vi "read command.vi"(9 "timeout ms (25000)":i32=25000) -> (0 "error out":errorcluster, 1 "command received":bool, 2 "command interface":T1={"command"=enum."Idle", "start time (ms)"=0, "Channel Indices"=[], "Scans per Sample"=1} {"Scans per Sample" min=1})   [LabVIEW 2012]
uses:
  DataServer/command cluster.ctl
  DataServer/command.ctl
panel:
  out "bytes read":dbl format="%.2f"
  out "byte received":bool
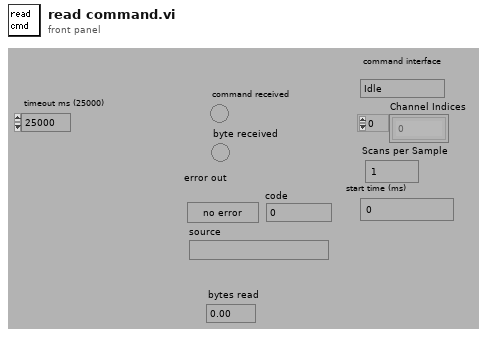
[diagram p1: front panel]
types:
  T1 = typedef "command cluster.ctl" = cluster{"command":T2, "start time (ms)":u32, "Channel Indices":i32[], "Scans per Sample":i32}
  T2 = typedef "command.ctl" = enum16{"Idle", "Send Data", "Send 1 Scan", "Logoff"}
  T3 = enum16{"clear", "add connection", "change command", "write state", "delete connection", "read"}
  T4 = enum16{"Standard", "Buffered", "CRLF", "Immediate"}
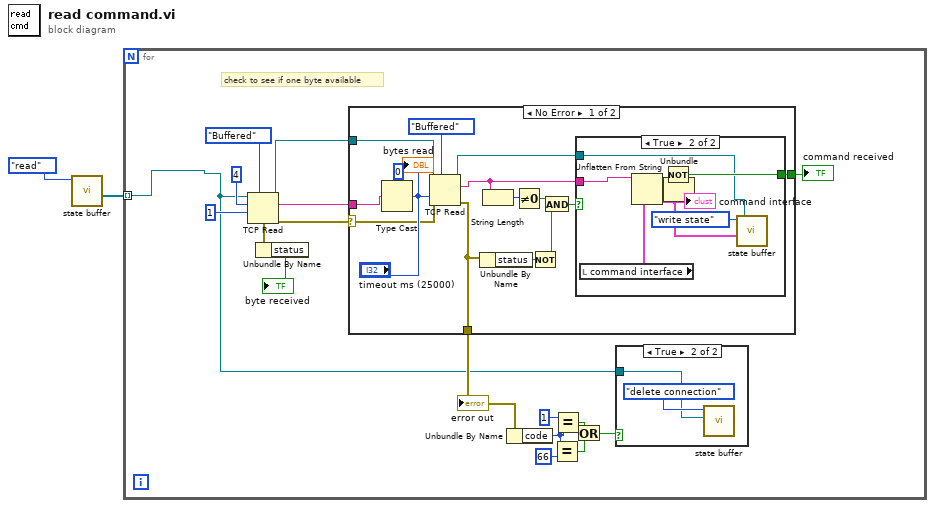
[diagram p0: block diagram]
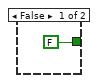
[diagram p3: hidden frame]
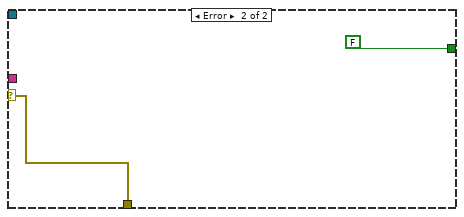
[diagram p4: hidden frame]
diagram:
  n1 = call "state buffer.vi"("command"=T3."read") -> ("connections"=w1:refnum<k5>[])  [unwired: 8 in, 2 out]
  n2 = for {
    tunnel: w1 -> [w4] mode=indexing
    # "check to see if one byte available"
    n3 = TCP Read(connection ID=w4, bytes to read=4, 7:T4."Buffered" ("mode (standard)"), 9:1) -> (connection ID out=w15:refnum<k5>, data out=w17:string, error out=w5:errorcluster)  [unwired: 1 in]
    n4 = Unbundle By Name(w5) -> ("status"=→"byte received":bool)
    n5 = case shown="No Error" w5 {
      selector: w5 -> [w22 w46]
      tunnel: w15 -> [w36 _]
      tunnel: w17 -> [w25 _]
      tunnel: [w23 w46] -> w12
      tunnel: [w27 FALSE] -> w14
      frame No Error {
        n6 = Type Cast(type=0, x=w25) -> (*(type *) &x=w26:i32)
        "bytes read" <- w26
        n7 = TCP Read(connection ID=w36, bytes to read=w26, error in (no error)=w22, 7:T4."Buffered" ("mode (standard)"), 9:"timeout ms (25000)") -> (connection ID out=w24:refnum<k5>, data out=w29:string, error out=w23:errorcluster)
        n8 = Unbundle By Name(w23) -> ("status"=w31:bool)
        n9 = String Length(string=w29) -> (length=w30:i32)
        n10 = Not Equal To 0?(x=w30) -> (x != 0?=w32:bool)
        n11 = Not(x=w31) -> (.not. x?=w33:bool)
        n12 = And(x=w32, y=w33) -> (x .and. y?=w28:bool)
        n13 = case shown="True" w28 {
          tunnel: w29 -> [_ w44]
          tunnel: [FALSE w42] -> w27
          tunnel: w24 -> [_ w40]
          frame False {
          }
          frame True {
            n14 = local read "command interface"() -> (w45:T1)
            n15 = Unflatten From String(type=w45, binary string=w44) -> (value=w39:T1, error out=w38:errorcluster)  [unwired: 3 in, 1 out]
            "command interface" <- w39
            n16 = Unbundle(w38) -> ("status"=w43:bool)  [unwired: 2 out]
            n17 = Not(x=w43) -> (.not. x?=w42:bool)
            n18 = call "state buffer.vi"("write state"=w39, "connection"=w40, "command"=T3."write state") -> ()  [unwired: 6 in, 3 out]
          }
        }
      }
      frame Error {
      }
    }
    "error out" <- w12
    "command received" <- w14
    n19 = Unbundle By Name(w12) -> ("code"=w11:i32)
    n20 = Equal?(x=w11, y=66) -> (x = y?=w8:bool)
    n21 = Equal?(x=1, y=w11) -> (x = y?=w9:bool)
    n22 = Or(x=w9, y=w8) -> (x .or. y?=w7:bool)
    n23 = case shown="True" w7 {
      tunnel: w4 -> [_ w19]
      frame False {
      }
      frame True {
        n24 = call "state buffer.vi"("connection"=w19, "command"=T3."delete connection") -> ()  [unwired: 7 in, 3 out]
      }
    }
  }
